vi "LWConexCC_Example.vi"() -> ()   [LabVIEW 2015]
uses:
  Newport.CONEXCC.CommandInterface
panel:
  out "VE error":i32
  out "errstring":string
  out "Information":string
  in  "Instrument Key":string
  out "error out":errorcluster
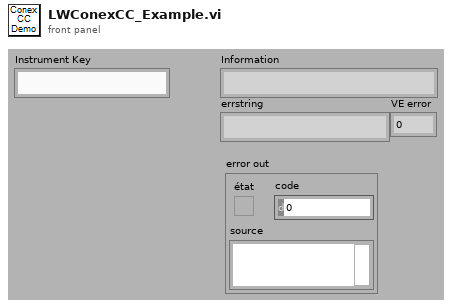
[diagram p1: front panel]
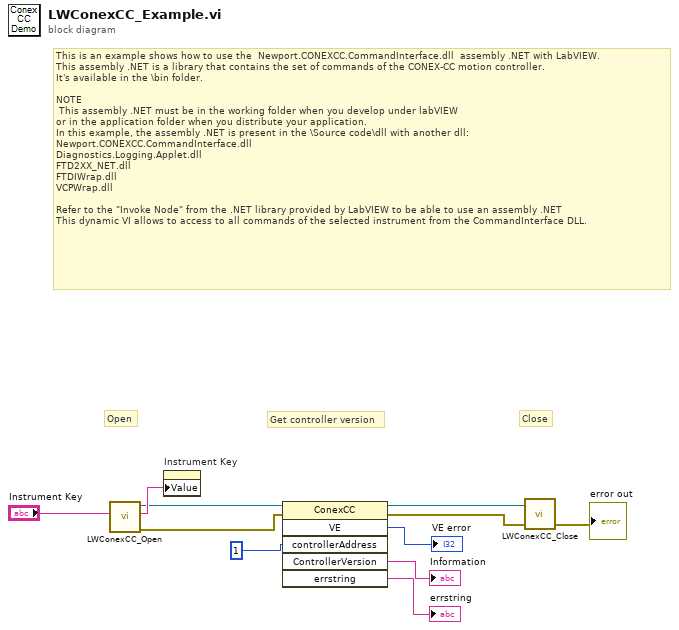
[diagram p0: block diagram]
diagram:
  # "This is an example shows how to use the  Newport.CONEXCC.CommandInterface.dll  assembly .NET with LabVIEW.\nThis assembly .NET is a library that contains the set of commands of the CONEX-CC motion controller. \nIt's available in the \\bin folder.\n\nNOTE\n This assembly .NET must be in the working folder when you develop under labVIEW \nor in the application folder when you distribute your application.\nIn this example, the assembly .NET is present in the \\Source code\\dll with another dll:\nNewport.CONEXCC.CommandInterface.dll\nDiagnostics.Logging.Applet.dll \nFTD2XX_NET.dll\nFTDIWrap.dll\nVCPWrap.dll\n\nRefer to the \"Invoke Node\" from the .NET library provided by LabVIEW to be able to use an assembly .NET\nThis dynamic VI allows to access to all commands of the selected instrument from the CommandInterface DLL."
  # "Get controller version"
  # "Close"
  # "Open"
  n1 = call "LWConexCC_Open.vi"("Instrument Key IN"="Instrument Key") -> ("error out"=w10:errorcluster, "Instrument Key OUT"=w8:string, "CommandInterfaceConexCC.ConexCC"=w7:refnum<k24>)  [unwired: 3 in, 1 out]
  n2 = property on="Instrument Key" class="Str"("Value"=w8) -> ()  [unwired: 2 in, 2 out]
  n3 = invoke class="ConexCC" method="VE"(reference=w7, error in=w10, "controllerAddress"=1) -> (reference out=w6:refnum<k24>, error out=w9:errorcluster, "VE"=→"VE error":i32, "ControllerVersion"=→"Information":string, "errstring"=→"errstring":string)  [unwired: 3 in, 1 out]
  n4 = call "LWConexCC_Close.vi"("error in (no error)"=w9, "CommandInterfaceConexCC.ConexCC"=w6) -> ("Error out"=→"error out":errorcluster)  [unwired: 3 in]
